vi "Initialize.vi"(7 "Serial Configuration":T1={"Baud Rate"=9600, "Parity"=0, "Data Bits"=8, "Stop Bits"=10} {"Stop Bits" items=["1.0"=10, "1.5"=15, "2.0"=20]; "Data Bits" items=["7"=7, "8"=8]; "Parity" items=["None", "Odd", "Even", "Mark", "Space"]; "Baud Rate" items=["300"=300, "600"=600, "1200"=1200, "2400"=2400, "4800"=4800, "9600"=9600, "19200"=19200]}, 8 "error in (no error)":errorcluster, 9 "Reset (True)":bool=TRUE, 10 "ID Query (True)":bool=TRUE, 11 "VISA resource name":refnum<visa-resource-name>) -> (0 "error out":errorcluster, 3 "VISA resource name out":refnum<visa-resource-name>)   [LabVIEW 2025]
doc: "Establishes communication with the instrument and optionally performs an instrument identification query and/or an instrument reset. It also places the instrument in a default state needed for other instrument driver operations. Therefore, call this VI before calling other instrument driver VIs for this instrument. Generally, you need to call the Initialize VI only once at the beginning of an application."
panel:
  # "(c) 2008 Andeen-Hagerling, Inc..  ALL RIGHTS RESERVED."
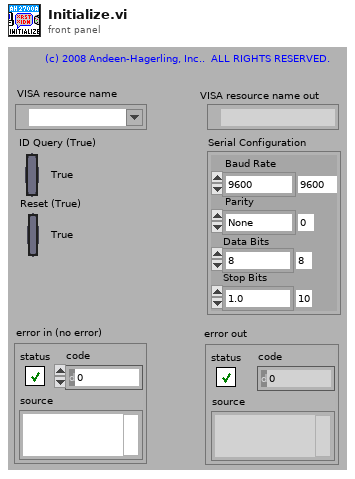
[diagram p1: front panel]
types:
  T1 = cluster{"Baud Rate":u32, "Parity":u16, "Data Bits":u16, "Stop Bits":u16}
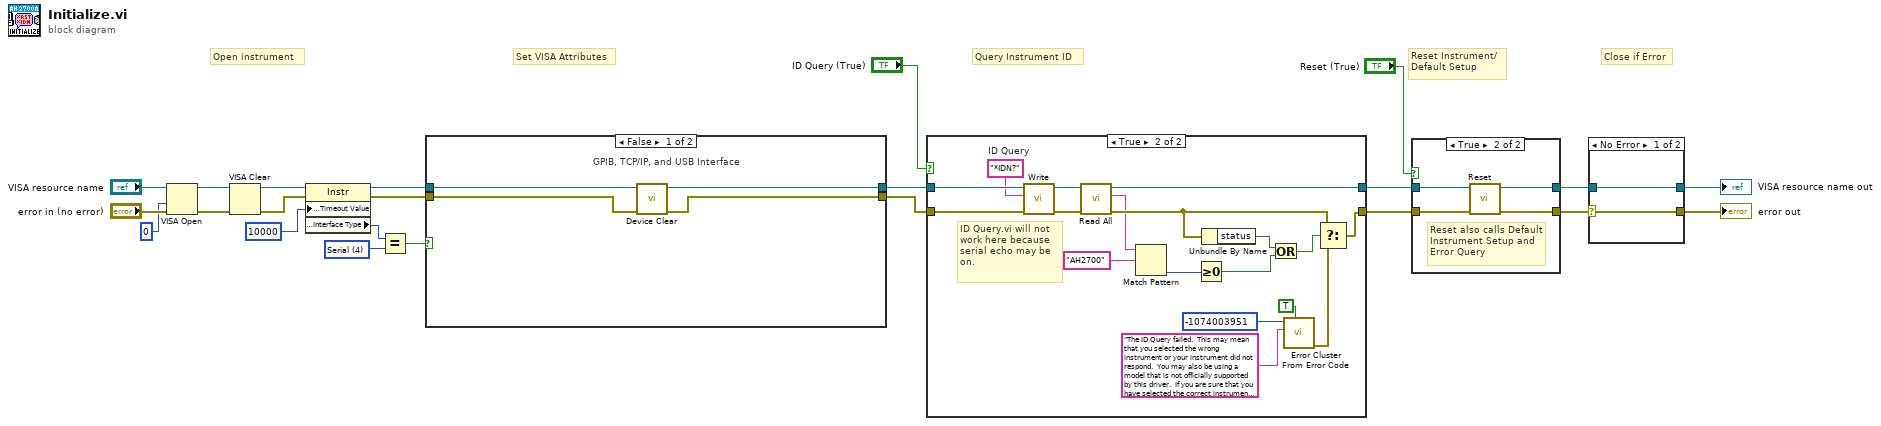
[diagram p0: block diagram]
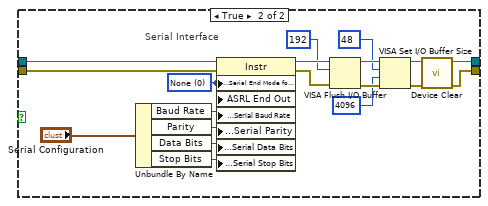
[diagram p2: hidden frame]
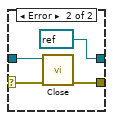
[diagram p3: hidden frame]
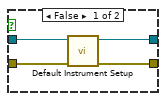
[diagram p4: hidden frame]
diagram:
  w10 = u16 4 items=["GPIB"=1, "VXI"=2, "GPIB-VXI"=3, "Serial"=4, "PXI"=5, "TCPIP"=6, "USB"=7] ("Interface Information:Interface Type")
  # "Set VISA Attributes"
  # "Close if Error"
  # "Query Instrument ID"
  # "Reset Instrument/\nDefault Setup"
  # "Open instrument"
  n1 = VISA Open(access mode=u32 0, error in (no error)="error in (no error)", VISA resource name="VISA resource name") -> (VISA resource name=w8:refnum<visa-resource-name>, error out=w7:errorcluster)  [unwired: 2 in]
  n2 = VISA Clear(VISA resource name=w8, error in (no error)=w7) -> (VISA resource name out=w6:refnum<visa-resource-name>, error out=w5:errorcluster)
  n3 = property class="Instr"(reference=w6, error in=w5, "General Settings:Timeout Value"=u32 10000) -> (reference out=w13:refnum<visa-resource-name>, error out=w12:errorcluster, "Interface Information:Interface Type"=w17:u16)
  n4 = Equal?(x=w17, y=w10) -> (x = y?=w11:bool)
  n5 = case shown="False" w11 {
    tunnel: [w24 w28] -> w15
    tunnel: [w25 w30] -> w14
    tunnel: w13 -> [w27 w45]
    tunnel: w12 -> [w26 w46]
    frame False {
      # "GPIB, TCP/IP, and USB Interface"
      n6 = call "Device Clear.vi"("error in"=w26, "VISA resource name"=w27) -> ("error out"=w25:errorcluster, "VISA resource name out"=w24:refnum<visa-resource-name>)  [unwired: 8 in]
    }
    frame True {
      w32 = u16 0 items=["None", "LastBit", "TermChar"] ("Serial Settings:Serial End Mode for Reads")
      # "Serial Interface"
      n7 = Unbundle By Name("Serial Configuration") -> ("Baud Rate"=w33:u32, "Parity"=w36:u16, "Data Bits"=w37:u16, "Stop Bits"=w34:u16)
      n8 = property class="Instr"(reference=w45, error in=w46, "Serial Settings:Serial End Mode for Reads"=w32, "ASRL End Out"=w32, "Serial Settings:Serial Baud Rate"=w33, "Serial Settings:Serial Parity"=w36, "Serial Settings:Serial Data Bits"=w37, "Serial Settings:Serial Stop Bits"=w34) -> (reference out=w41:refnum<visa-resource-name>, error out=w43:errorcluster)
      n9 = VISA Flush I/O Buffer(VISA resource name=w41, mask (16)=u16 192, error in (no error)=w43) -> (VISA resource name out=w44:refnum<visa-resource-name>, error out=w42:errorcluster)
      n10 = VISA Set I/O Buffer Size(VISA resource name=w44, mask (16)=u16 48, size (4096)=u32 4096 ("size (0)"), error in (no error)=w42) -> (VISA resource name out=w29:refnum<visa-resource-name>, error out=w31:errorcluster)
      n11 = call "Device Clear.vi"("error in"=w31, "VISA resource name"=w29) -> ("error out"=w30:errorcluster, "VISA resource name out"=w28:refnum<visa-resource-name>)  [unwired: 8 in]
    }
  }
  n12 = case shown="True" "ID Query (True)" {
    tunnel: [w47 w66] -> w22
    tunnel: [w48 w55] -> w23
    tunnel: w15 -> [w48 w53]
    tunnel: w14 -> [w47 w51]
    frame False {
    }
    frame True {
      w52 = "*IDN?"  # ID Query
      # "ID Query.vi will not\nwork here because \nserial echo may be\non."
      n13 = call "Write.vi"("error in"=w51, "command"=w52, "VISA resource name"=w53) -> ("error out"=w50:errorcluster, "VISA resource name out"=w49:refnum<visa-resource-name>)  [unwired: 7 in]
      n14 = call "Read All.vi"("error in"=w50, "VISA resource name"=w49) -> ("error out"=w56:errorcluster, "Message"=w54:string, "VISA resource name out"=w55:refnum<visa-resource-name>)  [unwired: 6 in, 1 out]
      n15 = Match Pattern(string=w54, regular expression="AH2700") -> (offset past match=w60:i32)  [unwired: 1 in, 3 out]
      n16 = Greater Or Equal To 0?(x=w60) -> (x >= 0?=w58:bool)
      n17 = Unbundle By Name(w56) -> ("status"=w59:bool)
      n18 = Or(x=w59, y=w58) -> (x .or. y?=w57:bool)
      n19 = call <vilib>:"Error Cluster From Error Code.vi"("show call chain? (False)"=TRUE, "error message (\"\")"="The ID Query failed.  This may mean that you selected the wrong instrument or your instrument did not respond.  You may also be using a model that is not officially supported by this driver.  If you are sure that you have selected the correct instrument and it is responding, try disabling the ID Query." ("Source (VI Name)"), "error code (0)"=-1074003951 ("Code")) -> ("error out"=w64:errorcluster)  [unwired: 6 in]
      n20 = Select(t=w56, s=w57, f=w64) -> (s? t:f=w66:errorcluster)
    }
  }
  n21 = case shown="True" "Reset (True)" {
    tunnel: w22 -> [w69 w71]
    tunnel: [w67 w74] -> w1
    tunnel: w23 -> [w70 w72]
    tunnel: [w68 w73] -> w2
    frame False {
      n22 = call "Default Instrument Setup.vi"("error in (no error)"=w69, "VISA resource name"=w70) -> ("error out"=w67:errorcluster, "VISA resource name out"=w68:refnum<visa-resource-name>)  [unwired: 8 in]
    }
    frame True {
      # "Reset also calls Default Instrument Setup and Error Query"
      n23 = call "Reset.vi"("error in (no error)"=w71, "VISA resource name"=w72) -> ("error out"=w74:errorcluster, "VISA resource name out"=w73:refnum<visa-resource-name>)  [unwired: 8 in]
    }
  }
  n24 = case shown="No Error" w1 {
    selector: w1 -> [w75 w78]
    tunnel: w2 -> [w76 w79]
    tunnel: [w76 refnum<visa-resource-name> refnum ("VISA resource name out")] -> w4
    tunnel: [w75 w80] -> w3
    frame No Error {
    }
    frame Error {
      n25 = call "Close.vi"("error in (no error)"=w78, "VISA resource name"=w79) -> ("error out"=w80:errorcluster)  [unwired: 9 in]
    }
  }
  "VISA resource name out" <- w4
  "error out" <- w3
